vi "conveyor contol.vi"() -> ()   [LabVIEW 2016]
panel:
  out "?":bool
  out "?":bool
  out "?":bool
  out "started":bool
  in  "Reset":bool
  in  "?":bool
  in  "Selector":bool
  out "conveyor":dbl(slide) scale=0.0..100.0
  # "Start"
  # "Stop"
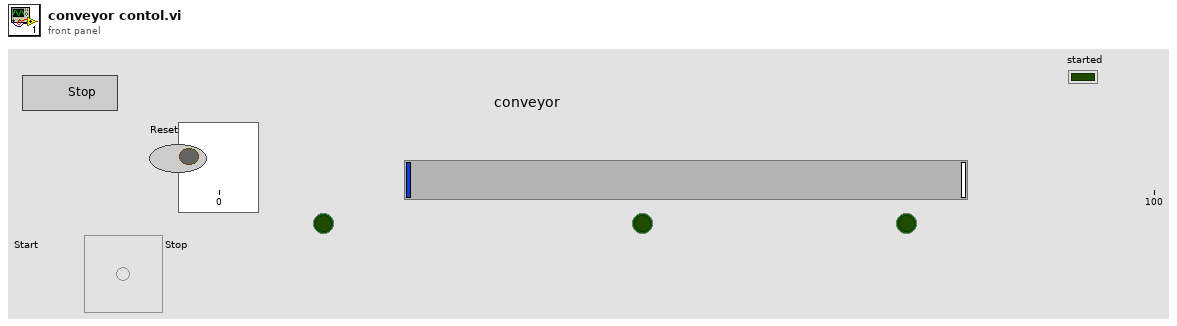
[diagram p1: front panel]
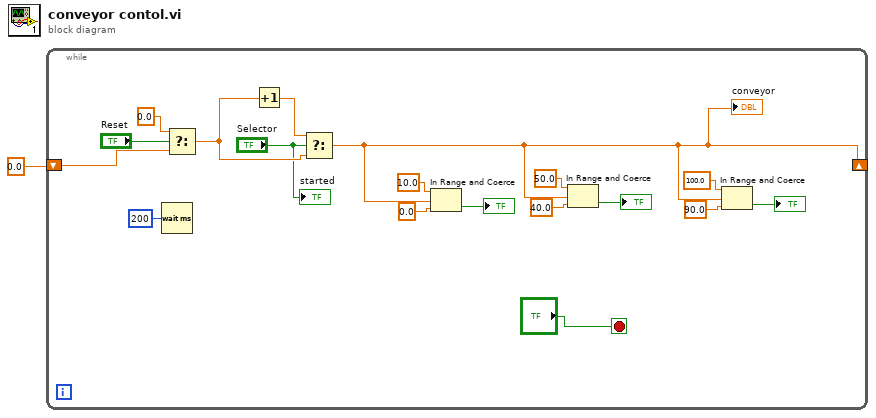
[diagram p0: block diagram]
diagram:
  n1 = while {
    shift-right: [w2] -> _
    shift-left: 0.0 -> [w17]
    stop <- "?" stop-if-true
    n2 = Wait (ms)(milliseconds to wait=u32 200) -> ()  [unwired: 1 out]
    n3 = Select(t=0.0, s="Reset", f=w17) -> (s? t:f=w14:dbl)
    n4 = Increment(x=w14) -> (x+1=w15:dbl)
    n5 = Select(t=w15, s="Selector", f=w14) -> (s? t:f=w2:dbl)
    "conveyor" <- w2
    n6 = In Range and Coerce(upper limit=10.0, x=w2, lower limit=0.0) -> (In Range?=→"?":bool)  [unwired: 1 out]
    n7 = In Range and Coerce(upper limit=50.0, x=w2, lower limit=40.0) -> (In Range?=→"?":bool)  [unwired: 1 out]
    n8 = In Range and Coerce(upper limit=100.0, x=w2, lower limit=90.0) -> (In Range?=→"?":bool)  [unwired: 1 out]
    "started" <- "Selector"
  }
